vi "Stepper Motor Controller Template for Students.vi"() -> ()   [LabVIEW 2013]
doc: "I. Description:\nThis example demonstrates how to output a continuous digital pattern on a digital IO board\n\nII. Instructions for Running:\n1. Select the Physical Channel to correspond to where your signal is output on the DAQ device.\n2. Specify the Rate of the output digital pattern.\n3. Enter the digital pattern data.\n4. You can change the output array on the fly. \n\nIII. Block Diagram Steps:\n1. Create an Digital Output Channel. \n2. Call the DAQmx (Sample Clock) VI which sets the sample clock rate. Additionally, set the sample mode to continuous.\n3. Write the data to the output buffer.\n4. Call the Start VI\n5. Loop continuously until the user presses the Stop button. Check for errors every 100 ms using the Is Task Done? VI\n6. Call the Clear Task VI to clear the Task.\n7. Use the popup dialog box to display an error or warning if any.\n\nIV. I/O Connections Overview:\nMake sure your signal output terminal matches the Physical Channel I/O Control. For further connection information, refer to your hardware reference manual."
uses:
  <vilib>/DAQmx/write.llb/DAQmx Write (Digital 1D U32 1Chan NSamp).vi
  <vilib>/DAQmx/create/channels.llb/DAQmx Create Channel (DO-Digital Output).vi
  <vilib>/DAQmx/configure/timing.llb/DAQmx Timing (Sample Clock).vi
  <vilib>/DAQmx/miscellaneous.llb/DAQmx Fill In Error Info.vi
panel:
  in  "Direction":u16(ring) items=["Clockwise", "Counter-Clockwise"]
  in  "Step":bool
  in  "Single/Continous Step":u16(ring)=1 items=["Finite Step", "Continuous Step"]
  in  "Step Type":u16(ring) items=["Single Step", "Power Step", "Half Step"]
  in  "stop":bool
  in  "Sample Clock Rate":dbl(slide)=305.35483870967744 scale=1.0..1000.0
  in  "Physical Channels":tag="Dev1/port0"
  # "74244 Chips acts as a buffer."
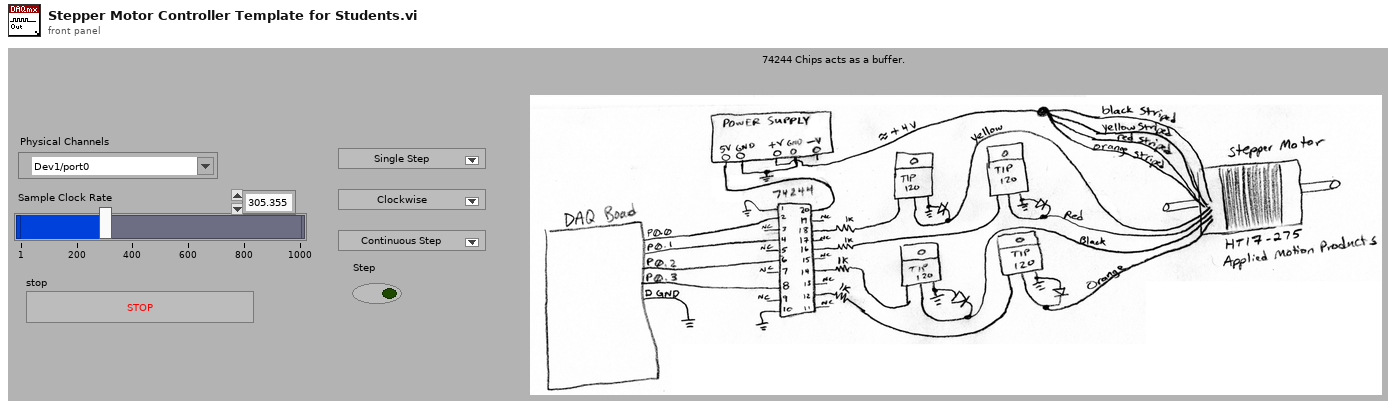
[diagram p1: front panel]
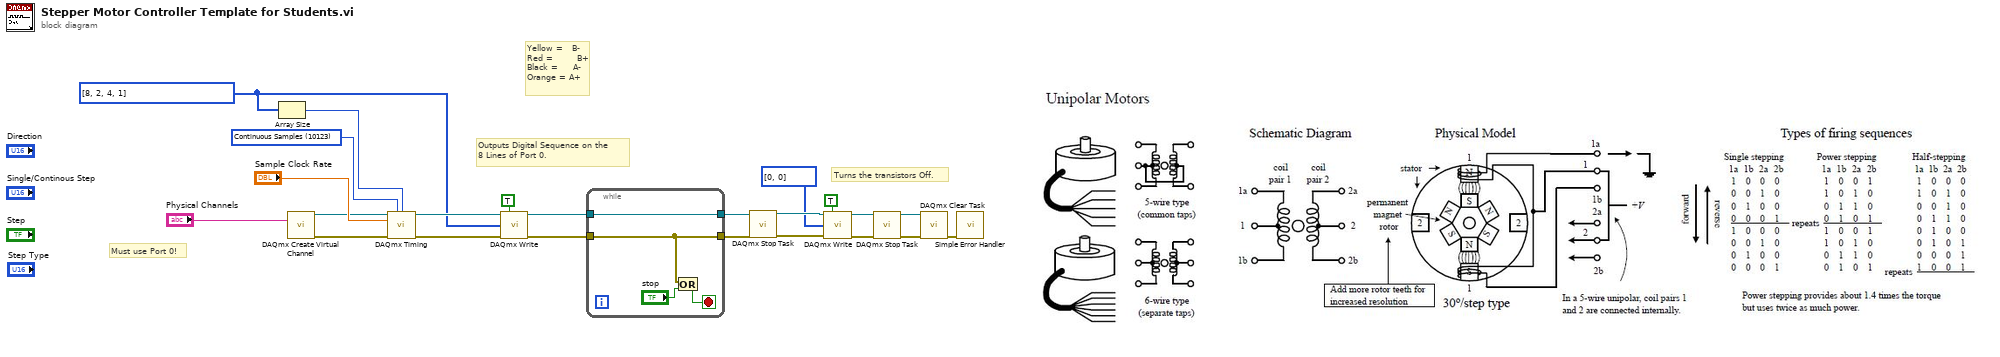
[diagram p0: block diagram]
diagram:
  w15 = u32[] [8, 2, 4, 1] ("data")
  w16 = 10123 items=["Finite Samples"=10178, "Continuous Samples"=10123] ("sample mode")
  # "Yellow =   B-\nRed =        B+\nBlack =     A-\nOrange = A+"
  # "Turns the transistors Off."
  # "Outputs Digital Sequence on the\n8 Lines of Port 0."
  # "Must use Port 0!"
  n1 = Array Size(array=w15) -> (size(s)=w19:i32)
  n2 = call-poly <vilib>:"DAQmx Create Virtual Channel.vi"("lines"="Physical Channels") -> ("task out"=w14:refnum<k21>, "error out"=w13:errorcluster)  [unwired: 13 in]
  n3 = call-poly <vilib>:"DAQmx Timing.vi"("task/channels in"=w14, "sample mode"=w16, "samples per channel"=w19, "rate"="Sample Clock Rate", "error in"=w13) -> ("task out"=w20:refnum<k21>, "error out"=w21:errorcluster)  [unwired: 9 in]
  n4 = call-poly <vilib>:"DAQmx Write.vi"("task/channels in"=w20, "auto start"=TRUE, "data"=w15, "error in"=w21) -> ("task out"=w11:refnum<k21>, "error out"=w12:errorcluster)  [unwired: 9 in, 1 out]
  n5 = while {
    tunnel: w12 -> [w24]
    tunnel: [w24] -> w8
    tunnel: [w27] -> w9
    tunnel: w11 -> [w27]
    stop <- w25 stop-if-true
    n6 = Or(x=w24, y="stop") -> (x .or. y?=w25:bool)
  }
  n7 = call <vilib>:"DAQmx Stop Task.vi"("task/channels in"=w9, "error in"=w8) -> ("task out"=w7:refnum<k21>, "error out"=w6:errorcluster)  [unwired: 12 in]
  n8 = call-poly <vilib>:"DAQmx Write.vi"("task/channels in"=w7, "auto start"=TRUE, "data"=u32[] [0, 0], "error in"=w6) -> ("task out"=w2:refnum<k21>, "error out"=w1:errorcluster)  [unwired: 9 in, 1 out]
  n9 = call <vilib>:"DAQmx Stop Task.vi"("task/channels in"=w2, "error in"=w1) -> ("task out"=w4:refnum<k21>, "error out"=w3:errorcluster)  [unwired: 12 in]
  n10 = call <vilib>:"DAQmx Clear Task.vi"("task in"=w4, "error in"=w3) -> ("error out"=w22:errorcluster)  [unwired: 13 in]
  n11 = call <vilib>:"Simple Error Handler.vi"("error in (no error)"=w22) -> ()  [unwired: 4 in, 5 out]
